vi "FRCts20_Backend_Test_Team_PUT.vi"(8 "error in (no error)":errorcluster, 11 "Team In":T1) -> (0 "error out":errorcluster, 1 "Time (ms)":u32, 2 "Status":string, 3 "Team Out":T1, 5 "Success":bool)   [LabVIEW 2013, in "FRCts20_Backend_TestCode.lvlib"]
uses:
  FRCts20_Backend_TestCode.lvlib
  FRCts20_Backend_API/FRCts20_Backend_API_Team.ctl
  FRCts20_Backend_API/FRCts20_Backend_API_SW.ctl
  FRCts20_Backend_API/FRCts20_Backend_API_Status.ctl
  FRCts20_Backend_API/FRCts20_Backend_API_Command_Team.ctl
  FRCts20_Backend_API/FRCts20_Backend_API_Team.vi
  FRCts20_Backend_API/FRCts20_Backend_API.lvlib
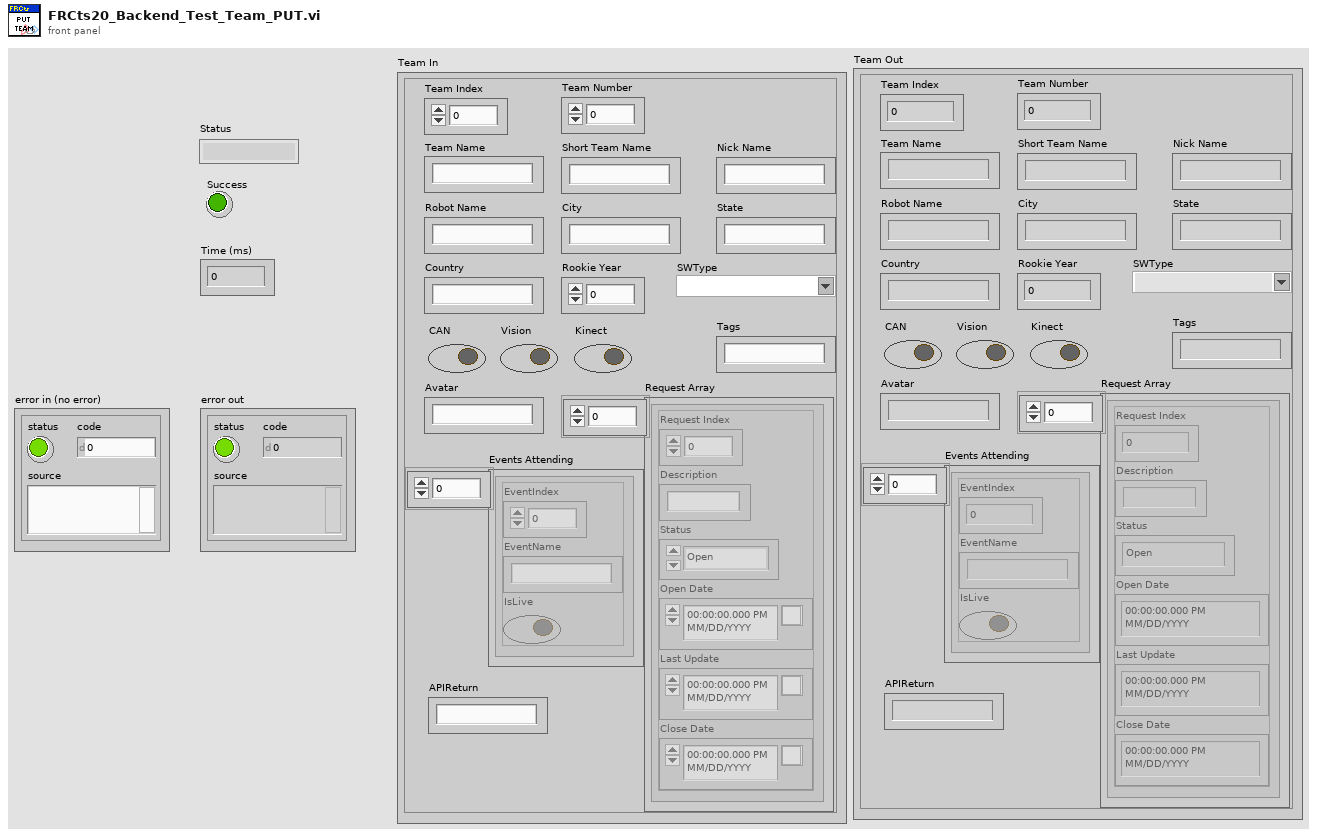
[diagram p1: front panel]
types:
  T1 = typedef "FRCts20_Backend_API.lvlib/FRCts20_Backend_API_Team.ctl" = cluster{"Team Index":u32, "Team Number":u32, "Team Name":string, "Short Team Name":string, "Nick Name":string, "Robot Name":string, "City":string, "State":string, "Country":string, "Rookie Year":u32, "SWType":T2, "CAN":bool, "Vision":bool, "Kinect":bool, "Tags":string, "Avatar":string, "Request Array":cluster{"Request Index":u32, "Description":string, "Status":T3, "Open Date":timestamp, "Last Update":timestamp, "Close Date":timestamp}[], "Events Attending":cluster{"EventIndex":dbl, "EventName":string, "IsLive":bool}[], "APIReturn":string}
  T2 = typedef "FRCts20_Backend_API.lvlib/FRCts20_Backend_API_SW.ctl" = string
  T3 = typedef "FRCts20_Backend_API.lvlib/FRCts20_Backend_API_Status.ctl" = enum16{"Open", "In Work", "Closed"}
  T4 = typedef "FRCts20_Backend_API.lvlib/FRCts20_Backend_API_Command_Team.ctl" = string
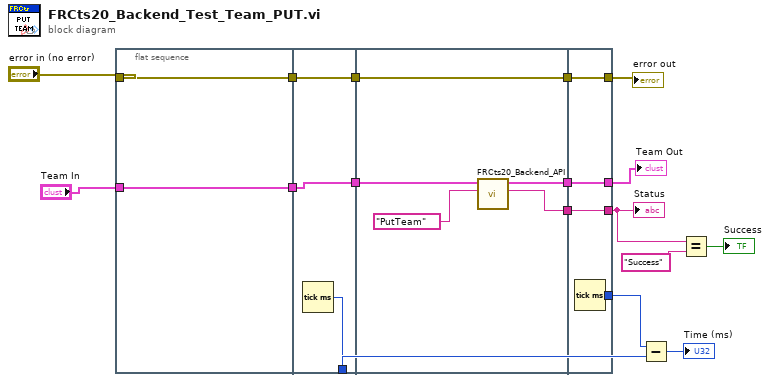
[diagram p0: block diagram]
diagram:
  n1 = flat-sequence {
    tunnel: "error in (no error)" -> [w19]
    tunnel: [w19] -> w17
    tunnel: [w18] -> w4
    tunnel: "Team In" -> [w18]
    tunnel: [w22] -> w7
    tunnel: [w21] -> w16
    tunnel: w17 -> [w21]
    tunnel: w4 -> [w20]
    tunnel: [w20] -> w2
    tunnel: [w27] -> w15
    tunnel: w16 -> [w27]
    tunnel: [w26] -> w14
    tunnel: [w25] -> w5
    tunnel: w2 -> [w24]
    tunnel: [w31] -> w8
    tunnel: [w30] -> w10
    tunnel: w15 -> [w30]
    tunnel: [w29] -> w6
    tunnel: w14 -> [w29]
    tunnel: [w28] -> w1
    tunnel: w5 -> [w28]
    frame #0 {
    }
    frame #1 {
      n2 = Tick Count (ms)() -> (millisecond timer value=w22:u32)
    }
    frame #2 {
      n3 = call-poly "FRCts20_Backend_API.vi"("Command"=T4 "PutTeam", "Team In"=w24) -> ("Status"=w26:string, "Team Out"=w25:T1)  [unwired: 7 in, 1 out]
    }
    frame #3 {
      n4 = Tick Count (ms)() -> (millisecond timer value=w31:u32)
    }
  }
  n5 = Subtract(x=w8, y=w7) -> (x-y=→"Time (ms)":u32)
  n6 = Equal?(x=w6, y="Success") -> (x = y?=→"Success":bool)
  "Status" <- w6
  "error out" <- w10
  "Team Out" <- w1
